vi "Strommessung.vi"(5 "Spannung":dbl) -> (0 "Prozentualladung (unngenau)":dbl, 1 "Amperesekunde verbraucht":dbl=-149.04557758721205, 2 "Wattsekunde verbraucht":dbl=-149.04557758721205, 3 "Strom mit Abweichungen":dbl=-149.04557758721205)   [LabVIEW 2016]
uses:
  <vilib>/myRIO/Instrument Drivers/Onboard IO/AI/typedefs/AI Reference.ctl
  <vilib>/myRIO/Common/Instrument Driver Framework/Utilities/typedefs/myRIO Generic Hardware Reference.ctl
  <vilib>/myRIO/Common/Instrument Driver Framework/Utilities/typedefs/Hardware Version Enum.ctl
  <vilib>/myRIO/Common/Instrument Driver Framework/Utilities/typedefs/myRIO v1.0 Reference.ctl
  <vilib>/myRIO/Common/Instrument Driver Framework/Utilities/typedefs/Generic FPGA Reference.ctl
  <vilib>/myRIO/Common/Instrument Driver Framework/myRIO v1.0/AI/typedefs/AI Channels List.ctl
  <vilib>/myRIO/Common/Instrument Driver Framework/myRIO v1.0/AI/typedefs/AI Channels Enum.ctl
  <vilib>/myRIO/Common/Instrument Driver Framework/Utilities/typedefs/Analog Scaling Constants List.ctl
  <vilib>/myRIO/Common/Instrument Driver Framework/Utilities/typedefs/Analog Scaling Constants.ctl
  <vilib>/userdefined/High Color/nirio_resource_hc.ctl
  <vilib>/myRIO/Common/Instrument Driver Framework/Utilities/vis/Is FPGA Ref Available.vi
  <vilib>/myRIO/Common/Instrument Driver Framework/myRIO v1.0/AI/vis/myRIO v1.1 Open AI.vi
  <vilib>/myRIO/Instrument Drivers/Onboard IO/AI/vis/Read.vi
  <vilib>/myRIO/Common/Instrument Driver Framework/Utilities/vis/Validate Channels.vi
  <vilib>/myRIO/Common/Instrument Driver Framework/myRIO v1.0/AI/vis/myRIO v1.0 Reserve AI.vi
  <vilib>/myRIO/Common/Instrument Driver Framework/myRIO v1.0/AI/vis/myRIO v1.0 Build MUX Configuration AI.vi
  <vilib>/myRIO/Common/Instrument Driver Framework/myRIO v1.0/Resource Manager/vis/myRIO v1.0 Reserve Channel List.vi
  <vilib>/myRIO/Common/Instrument Driver Framework/myRIO v1.0/Resource Manager/vis/myRIO v1.0 Reserve Channel.vi
  <vilib>/myRIO/Common/Instrument Driver Framework/myRIO v1.0/Resource Manager/vis/myRIO v1.0 Unreserve Channel.vi
  <vilib>/myRIO/Common/Instrument Driver Framework/myRIO v1.0/Resource Manager/vis/myRIO v1.0 Build Mutex Name.vi
  <vilib>/Utility/VariantDataType/GetNumericInfo.vi
  <vilib>/Utility/error.llb/Error Cluster From Error Code.vi
  <vilib>/myRIO/Common/Instrument Driver Framework/myRIO v1.0/myRIO v1.1 Open.vi
  <vilib>/myRIO/Common/Instrument Driver Framework/myRIO v1.0/AI/vis/myRIO v1.0 Get Scaling Constants AI.vi
  <vilib>/myRIO/Common/Instrument Driver Framework/Utilities/vis/IO Manager.vi
  <vilib>/myRIO/Common/Instrument Driver Framework/Utilities/vis/Configuration Manager.vi
  <vilib>/myRIO/Common/Instrument Driver Framework/myRIO v1.0/myRIO v1.0 Close.vi
  <vilib>/myRIO/Common/Instrument Driver Framework/myRIO v1.0/AI/vis/myRIO v1.0 Read AI.vi
  <vilib>/myRIO/Express VI/Onboard IO/AI/AI Express VI.xnode
  <vilib>/myRIO/Instrument Drivers/Onboard IO/AI/vis/myRIO AI Open.xnode
  <vilib>/myRIO/Instrument Drivers/Onboard IO/AI/AI.lvlib
panel:
  out "Strom ohne Abweichung":dbl=-149.04557758721205
  out "Wahre Abweichung Mittelwert":dbl=-149.04557758721205
  out "Standartabweichung Strom\n+ -":dbl=-149.04557758721205
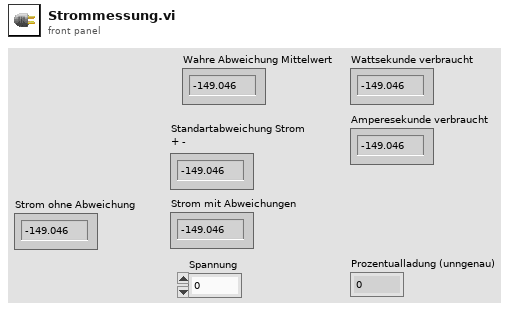
[diagram p1: front panel]
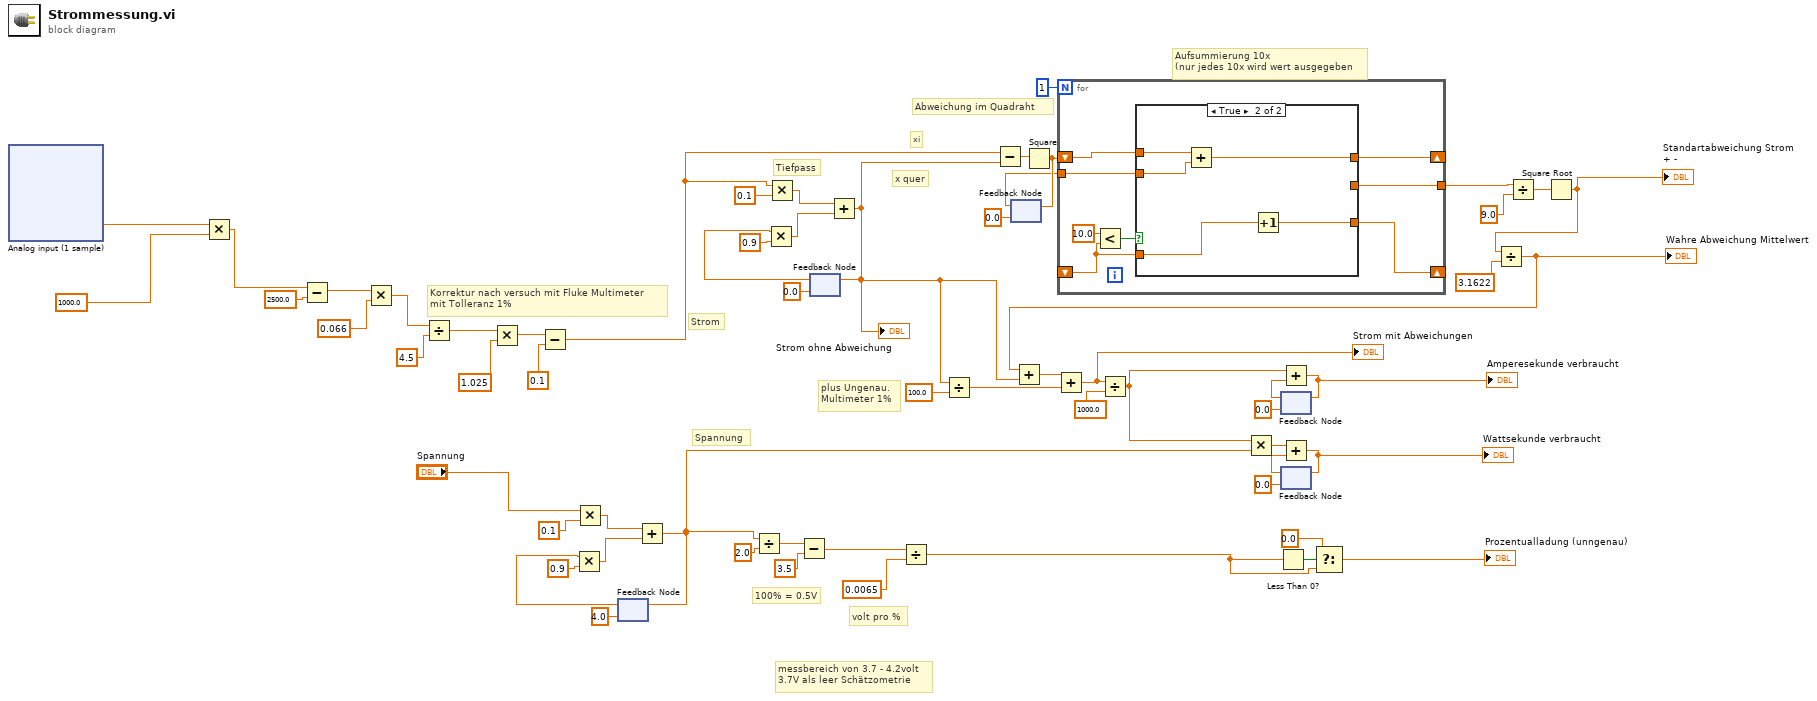
[diagram p0: block diagram]
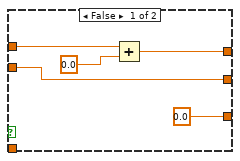
[diagram p2: hidden frame]
diagram:
  # "Spannung"
  # "Strom"
  # "Aufsummierung 10x\n(nur jedes 10x wird wert ausgegeben"
  # "plus Ungenau.\nMultimeter 1%"
  # "xi"
  # "x quer"
  # "Abweichung im Quadraht"
  # "Tiefpass"
  # "100% = 0.5V"
  # "messbereich von 3.7 - 4.2volt\n3.7V als leer Schätzometrie"
  # "volt pro %"
  # "Korrektur nach versuch mit Fluke Multimeter\nmit Tolleranz 1%"
  n1 = xnode "Analog input (1 sample)"() -> ("C/AI1 (AI1)"=w54:dbl)  [unwired: 1 in, 1 out]
  n2 = Multiply(x=w54, y=1000.0) -> (x*y=w59:dbl)
  n3 = Subtract(x=w59, y=2500.0) -> (x-y=w57:dbl)
  n4 = Multiply(x=w57, y=0.066) -> (x*y=w51:dbl)
  n5 = Divide(x=w51, y=4.5 ("x")) -> (x/y=w50:dbl)
  n6 = Multiply(x=w50, y=1.025) -> (x*y=w46:dbl)
  n7 = Subtract(x=w46, y=0.1) -> (x-y=w7:dbl)
  n8 = Multiply(x="Spannung", y=0.1) -> (x*y=w37:dbl)
  n9 = feedback #1(4.0) -> (w35:dbl)
  n10 = Multiply(x=w35, y=0.9) -> (x*y=w40:dbl)
  n11 = Add(x=w37, y=w40) -> (x+y=w25:dbl)
  n12 = feedback-in #1(w25) -> ()
  n13 = Divide(x=w25, y=2.0) -> (x/y=w30:dbl)
  n14 = Multiply(x=w7, y=0.1) -> (x*y=w47:dbl)
  n15 = Subtract(x=w30, y=3.5) -> (x-y=w28:dbl)
  n16 = feedback #2(0.0) -> (w53:dbl)
  n17 = Multiply(x=w53, y=0.9) -> (x*y=w61:dbl)
  n18 = Add(x=w47, y=w61) -> (x+y=w6:dbl)
  "Strom ohne Abweichung" <- w6
  n19 = feedback-in #2(w6) -> ()
  n20 = Divide(x=w28, y=0.0065) -> (x/y=w26:dbl)
  n21 = Divide(x=w6, y=100.0) -> (x/y=w8:dbl)
  n22 = Subtract(x=w7, y=w6) -> (x-y=w21:dbl)
  n23 = feedback #3(0.0) -> (w14:dbl)
  n24 = Square(x=w21) -> (x^2=w15:dbl)
  n25 = feedback-in #3(w15) -> ()
  n26 = for {
    N: 1 -> [_]
    shift-right: [w68] -> _
    shift-left: w15 -> [w69]
    shift-right: [w67] -> _
    shift-left: _ -> [w64]
    tunnel: w14 -> [w63]
    tunnel: [w62] -> w13
    n27 = Less?(x=10.0, y=w64) -> (x < y?=w65:bool)
    n28 = case shown="True" w65 {
      tunnel: w69 -> [w71 w79]
      tunnel: [w72 w76] -> w68
      tunnel: [0.0 w78] -> w67
      tunnel: w64 -> [_ w77]
      tunnel: w63 -> [w70 w75]
      tunnel: [w70 _] -> w62
      frame False {
        n29 = Add(x=w71, y=0.0) -> (x+y=w72:dbl)
      }
      frame True {
        n30 = Add(x=w79, y=w75) -> (x+y=w76:dbl)
        n31 = Increment(x=w77) -> (x+1=w78:dbl)
      }
    }
  }
  n32 = Less Than 0?(x=w26) -> (x < 0?=w33:bool)
  n33 = feedback #4(0.0) -> (w42:dbl)
  n34 = feedback #5(0.0) -> (w23:dbl)
  n35 = Select(t=0.0, s=w33, f=w26) -> (s? t:f=→"Prozentualladung (unngenau)":dbl)
  n36 = Divide(x=w13, y=9.0) -> (x/y=w12:dbl)
  n37 = Square Root(x=w12) -> (sqrt(x)=w17:dbl)
  "Standartabweichung Strom\n+ -" <- w17
  n38 = Divide(x=w17, y=3.1622) -> (x/y=w11:dbl)
  "Wahre Abweichung Mittelwert" <- w11
  n39 = Add(x=w11, y=w6) -> (x+y=w10:dbl)
  n40 = Add(x=w10, y=w8) -> (x+y=w5:dbl)
  "Strom mit Abweichungen" <- w5
  n41 = Divide(x=w5, y=1000.0) -> (x/y=w3:dbl)
  n42 = Multiply(x=w3, y=w25) -> (x*y=w22:dbl)
  n43 = Add(x=w3, y=w42) -> (x+y=w1:dbl)
  "Amperesekunde verbraucht" <- w1
  n44 = feedback-in #4(w1) -> ()
  n45 = Add(x=w22, y=w23) -> (x+y=w2:dbl)
  "Wattsekunde verbraucht" <- w2
  n46 = feedback-in #5(w2) -> ()
